vi "Komm Modbus_F.vi"() -> (0 "error IO":errorcluster)   [LabVIEW 2020, in "ABB-EL3000.lvlib" / "FID.lvlib"]
uses:
  FID.lvlib
  Aktion FGV Modbus_F.ctl
  Stoerungen/Stoerungen Messgeraet/Aktionen Kommunikation Stoerung.ctl
  Stoerungen/Stoerungen.lvlib
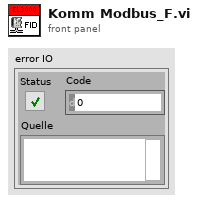
[diagram p1: front panel]
types:
  T1 = typedef "ABB-EL3000.lvlib/FID.lvlib/Aktion FGV Modbus_F.ctl" = enum16{"lesen", "Verbindung herstellen", "Verbindung trennen", "Komm"}
  T2 = typedef "Stoerungen.lvlib/Aktionen Kommunikation Stoerung.ctl" = enum16{"lesen", "init", "FT-IR Komm", "FT-IR Betriebsart", "FT-IR Hintergrund", "cRIO Komm", "PNS Komm", "Dichtheitstest", "Life Bit", "FTIR Komm AK", "PMA Komm", "FID Komm", "PMA Cal", "FID Ch4 Cal", "FID THC Cal", "Cal Timeout", "VFS 1 Komm", "VFS 2 Komm", "VFS 3 Komm", "VFS 4 Komm", "TRE 08 Komm", "CG-Test vorzeitig", "CG-Test Span 1", "CG-Test Span 2", "CG-Test Span 3", "CG-Test Messgas", "CG-Test löschen", "Test", "Amium AK", "AK Recept konfig", "AK Name konfig", "AK EKFG konfig"}
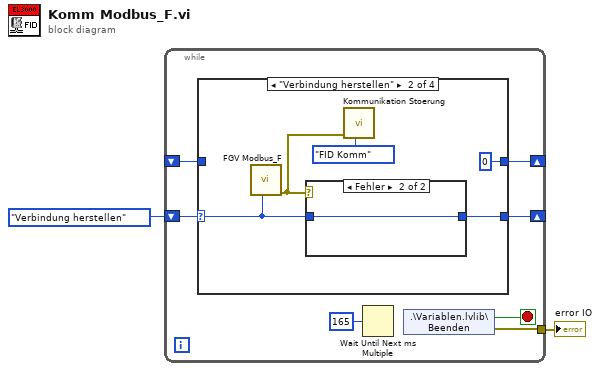
[diagram p0: block diagram]
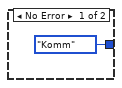
[diagram p3: hidden frame]
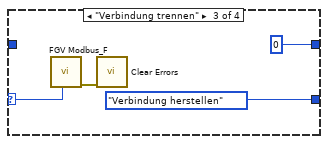
[diagram p4: hidden frame]
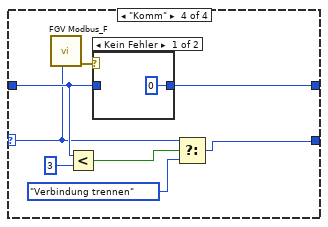
[diagram p5: hidden frame]
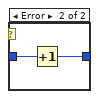
[diagram p6: hidden frame]
diagram:
  n1 = while {
    shift-right: [w9] -> _
    shift-left: Aktion_FGV_Modbus_F."Verbindung herstellen" ("Aktion") -> [w8]
    tunnel: [w5] -> w1
    shift-right: [w4] -> _
    shift-left: _ -> [w3]
    stop <- w6 stop-if-true
    n2 = case shown="\"Verbindung herstellen\"" w8 {
      selector: w8 -> [w11 w16 w22 w25]
      tunnel: [w11 w15 Aktion_FGV_Modbus_F."Verbindung herstellen" ("Aktion") w23] -> w9
      tunnel: [w10 0 0 w29] -> w4
      tunnel: w3 -> [w10 _ _ w28]
      frame "lesen", Default {
      }
      frame "Verbindung herstellen" {
        n3 = call "FGV Modbus_F.vi"("Aktion"=w16) -> ("error out"=w12:errorcluster)  [unwired: 10 in]
        n4 = case shown="Fehler" w12 {
          tunnel: w16 -> [_ w18]
          tunnel: [Aktion_FGV_Modbus_F."Komm" ("Aktion") w18] -> w15
          frame No Error {
          }
          frame Error {
          }
        }
        n5 = call "Kommunikation Stoerung.vi"("Aktionen"=Aktionen_Kommunikation_Stoerung."FID Komm", "error in"=w12) -> ()  [unwired: 9 in, 1 out]
      }
      frame "Verbindung trennen" {
        n6 = call "FGV Modbus_F.vi"("Aktion"=w22) -> ("error out"=w20:errorcluster)  [unwired: 10 in]
        n7 = call <vilib>:"Clear Errors.vi"("error in (no error)"=w20) -> ()  [unwired: 5 in, 2 out]
      }
      frame "Komm" {
        n8 = call "FGV Modbus_F.vi"("Aktion"=w25) -> ("error out"=w30:errorcluster)  [unwired: 10 in]
        n9 = Less?(x=w28, y=3) -> (x < y?=w26:bool)
        n10 = case shown="Kein Fehler" w30 {
          tunnel: w28 -> [_ w33]
          tunnel: [0 w32] -> w29
          frame No Error {
          }
          frame Error {
            n11 = Increment(x=w33) -> (x+1=w32:i32)
          }
        }
        n12 = Select(t=w25, s=w26, f=Aktion_FGV_Modbus_F."Verbindung trennen" ("Aktion")) -> (s? t:f=w23:T1)
      }
    }
    n13 = Wait Until Next ms Multiple(millisecond multiple=u32 165 ("Vielfache von ms")) -> ()  [unwired: 1 out]
    n14 = shared-variable ".\\Variablen.lvlib\\Beenden"() -> (w6:bool, error out=w5:errorcluster)  [unwired: 1 in]
  }
  "error IO" <- w1
